vi "main.vi"() -> ()   [LabVIEW 2021]
uses:
  DIAS_Pyrometer/DIAS_Pyrometer.lvlib
  typedefs/MachineStates.ctl
  typedefs/GUIMsg.ctl
  7af14925-e625-4b71-82b2-5c041dc11c26.vi
  DIAS_Pyrometer/VIs/Server/TimeResp.ctl
  DIAS_Pyrometer/VIs/Server/PyrospotDat.ctl
  Library/TerminalDef.ctl
  Library/LibDan.lvlib
  Library/PromptWrite.vi
  Library/PassFailWrite.vi
  95fd1d63-83c7-47ba-856f-b2f4cd3ba726.vi
  DIAS_Pyrometer/SetTResp.vi
  DIAS_Pyrometer/SetEmi.vi
  5cd4da98-0f3d-48f1-83bd-2073b8292d09.vi
  Library/ErrorWrite.vi
  ec44e22e-e0b8-4ec3-9cb0-dd0efa94501a.vi
  4efa8287-acc7-4af3-aaf1-ea9888832d28.vi
  34df0790-2c42-4b95-90d0-b75bcdfa5c96.vi
  f4e94fa1-7f87-4e7c-9be3-fe64689eeddf.vi
  d668ad43-4b8f-4c4d-b9d8-3098d740c719.vi
  ba4263dd-0b88-4781-9c96-c1ae58dad5df.vi
  <vilib>/Utility/config.llb/Config Data RefNum.ctl
  <vilib>/Utility/config.llb/NI_LVConfig.lvlib
panel:
  out "LED_Serving":bool
  out "LED_Connected":bool
  in  "Stop":bool
  in  "Server_But":bool
  in  "Connect_But":bool
  out "Terminal":string
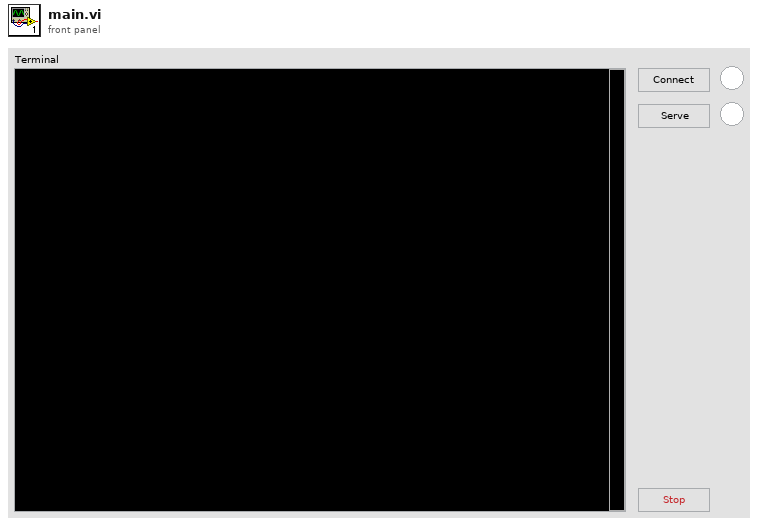
[diagram p1: front panel]
types:
  T1 = cluster{"Name":string, "Map":map{string, string}}
  T2 = typedef "DIAS_Pyrometer.lvlib/TimeResp.ctl" = u16
  T3 = typedef "LibDan.lvlib/TerminalDef.ctl" = cluster{"Terminal":cluster{"Data":string, "Prompt":string, "Output Refnum":refnum<vi>, "Input":string, "Input Refnum":refnum<vi>}, "TCP":cluster{"HostIP":string, "ServiceName":string, "Port":u16, "Timeout":i32, "TCP ID":refnum<k5>, "TCPConID":refnum<k5>, "Listening?":bool, "ClientCon?":bool}, "Config":cluster{"Path":path, "PathRef":T4, "NewFile?":bool, "Sections":cluster{"Name":string, "Map":map{string, string}}[]}}
  T4 = typedef "NI_LVConfig.lvlib/Config Data RefNum.ctl" = refnum<k1>
  T5 = typedef "DIAS_Pyrometer.lvlib/PyrospotDat.ctl" = cluster{"COM":u16, "Good":bool, "Address":i32, "Emissivity":sgl, "T95":T2, "Temp(K)":dbl, "Time":timestamp, "Laser":bool}
  T6 = typedef "MachineStates.ctl" = enum16{"NOP", "ProgInit", "PyroCon", "PyroDis", "Error", "SetPyro", "GetPyro", "ServerCon", "ServerDis", "ServeData", "ServerListen", "STOP"}
  T7 = typedef "GUIMsg.ctl" = cluster{T6, "exit?":bool}
  T8 = cluster{"Name":string, "Map":map{string, string}}[]
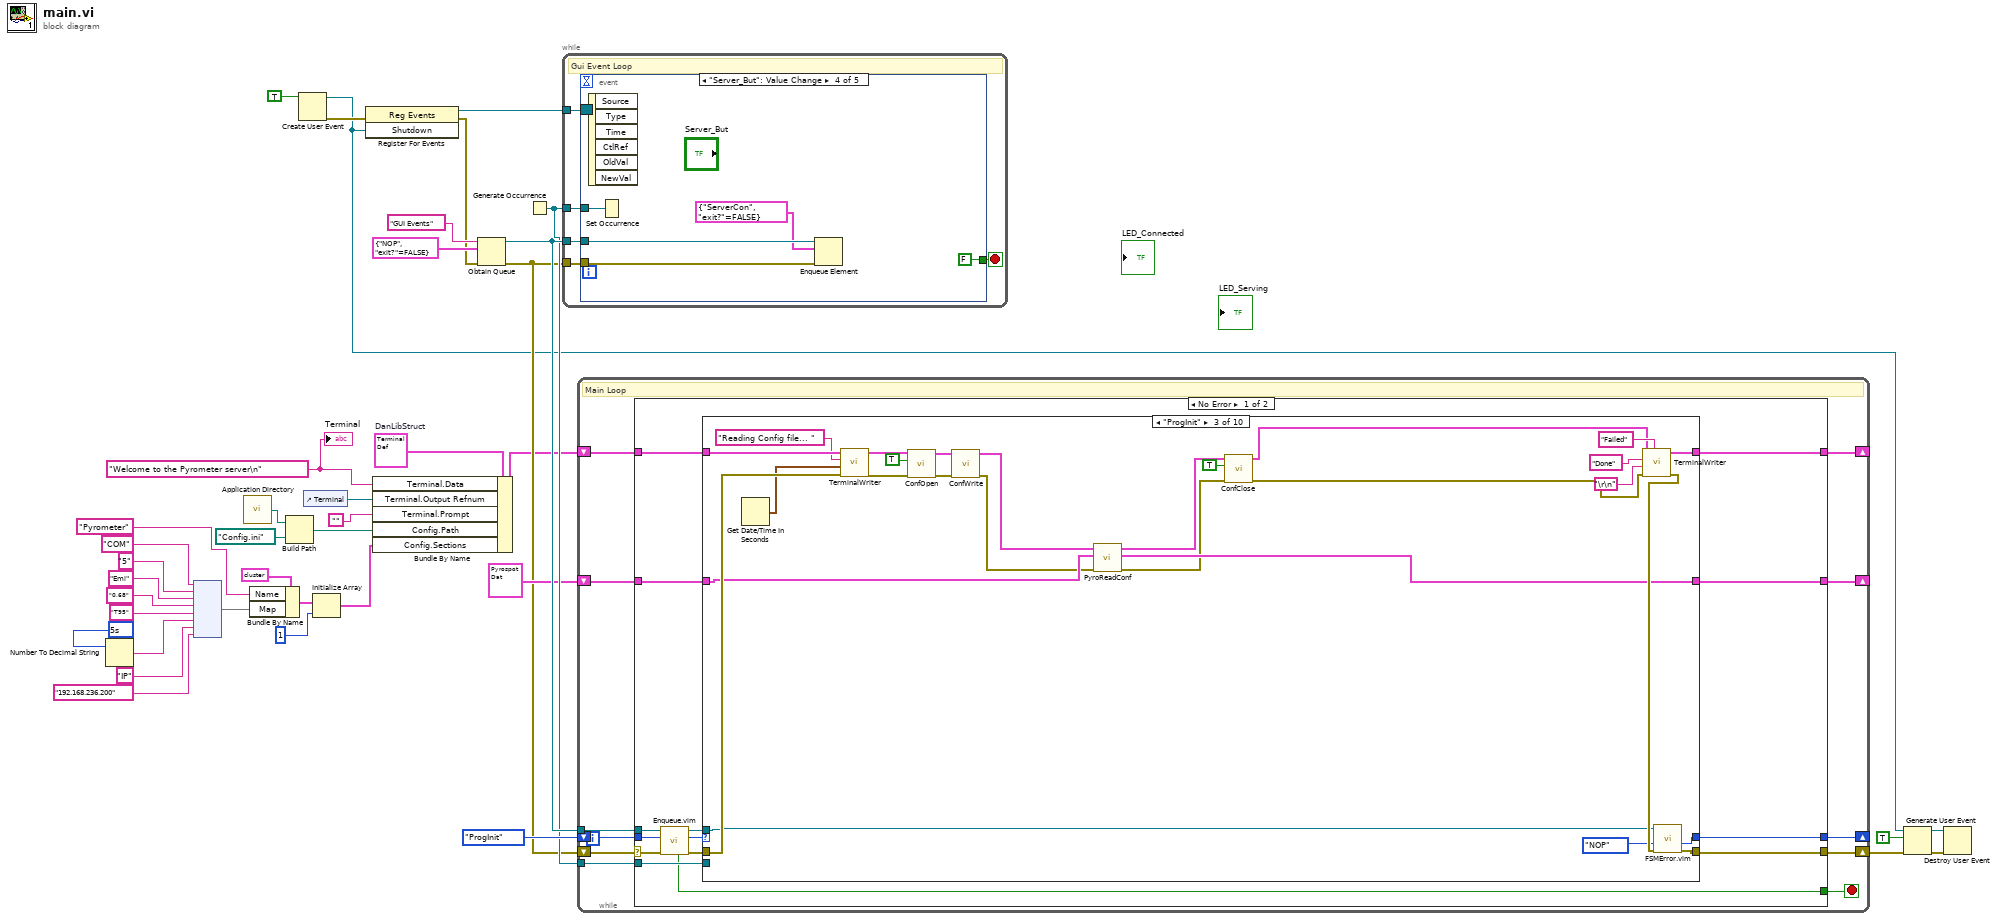
[diagram p0: block diagram]
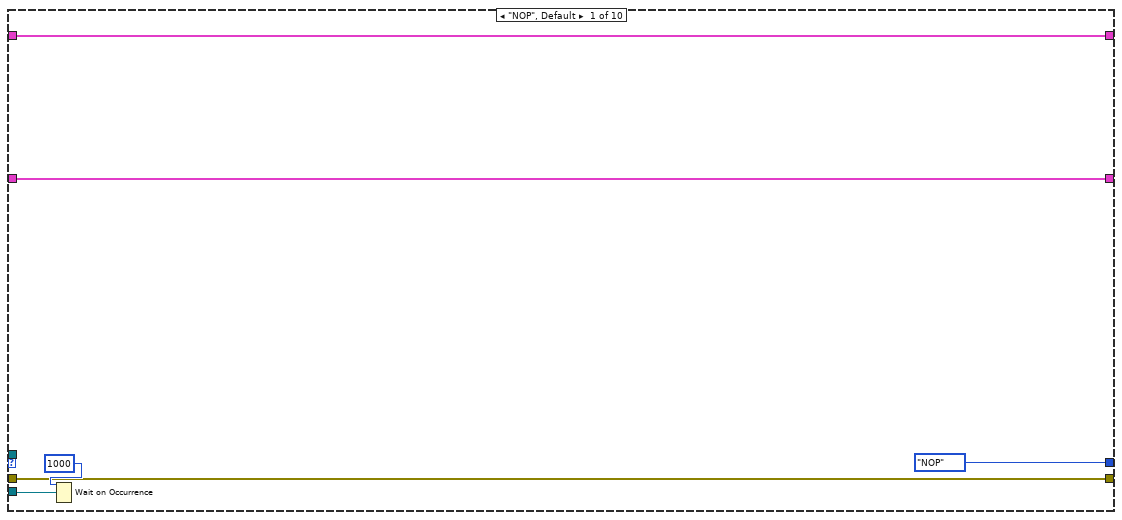
[diagram p2: hidden frame]
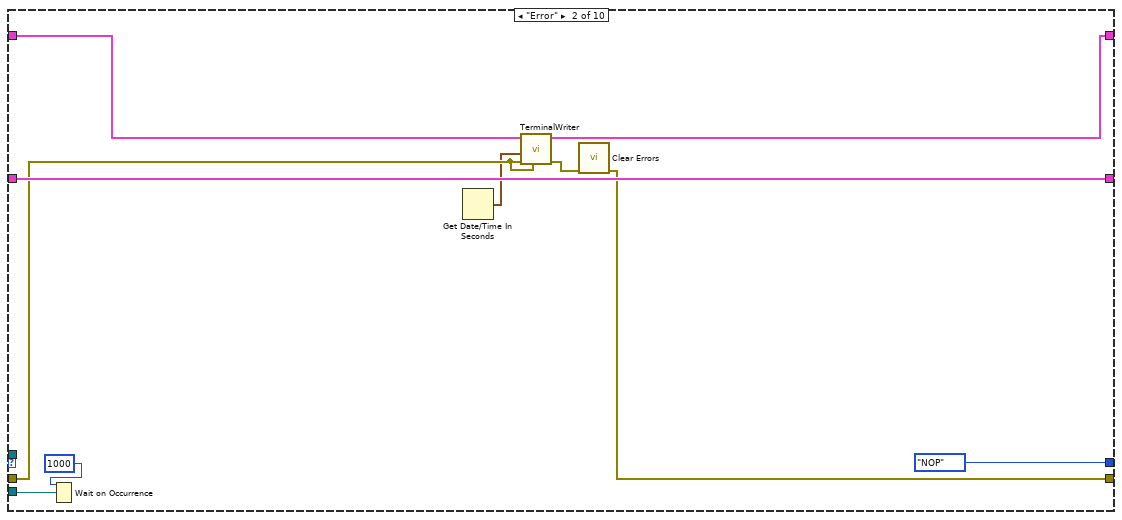
[diagram p3: hidden frame]
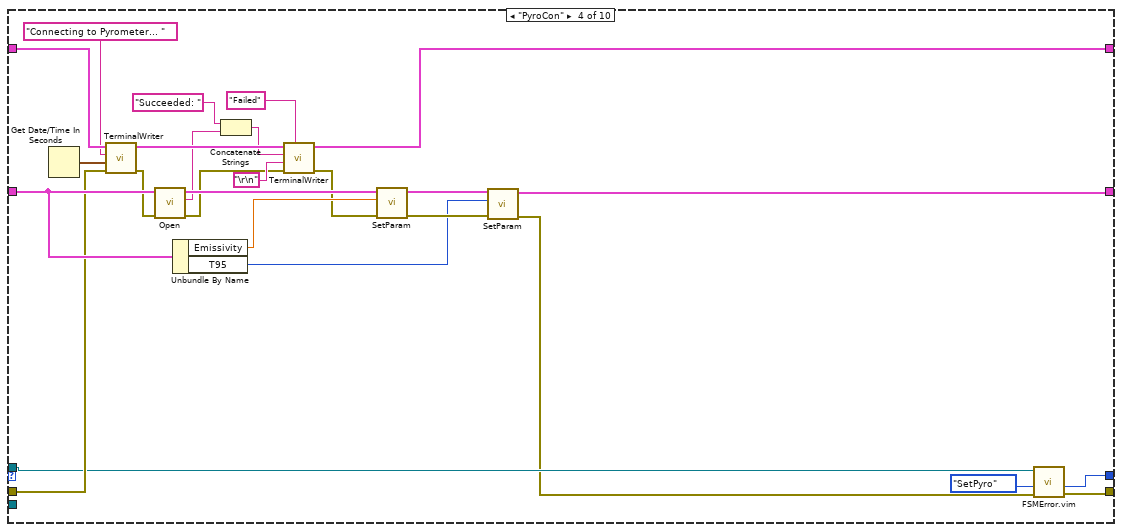
[diagram p4: hidden frame]
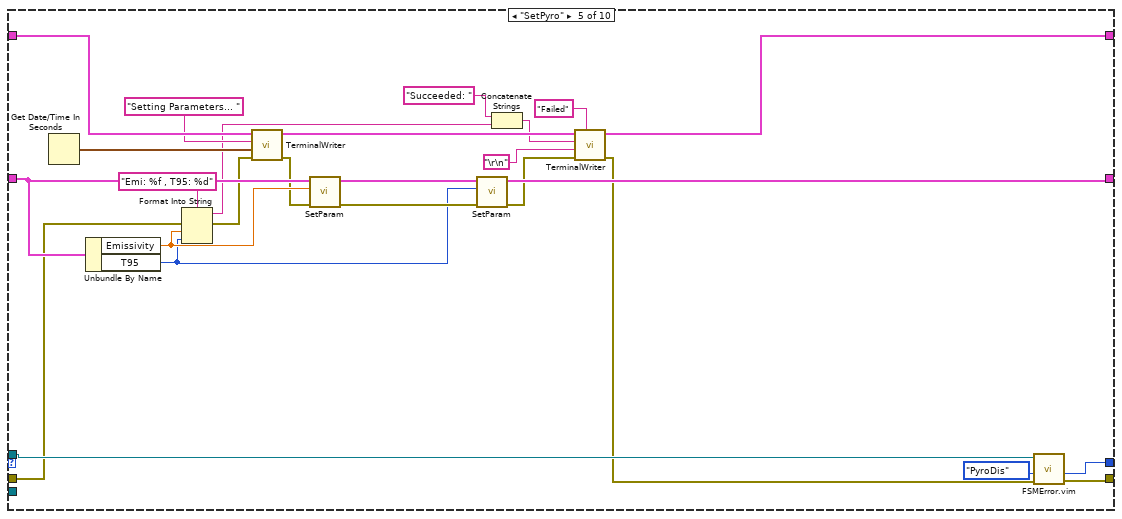
[diagram p5: hidden frame]
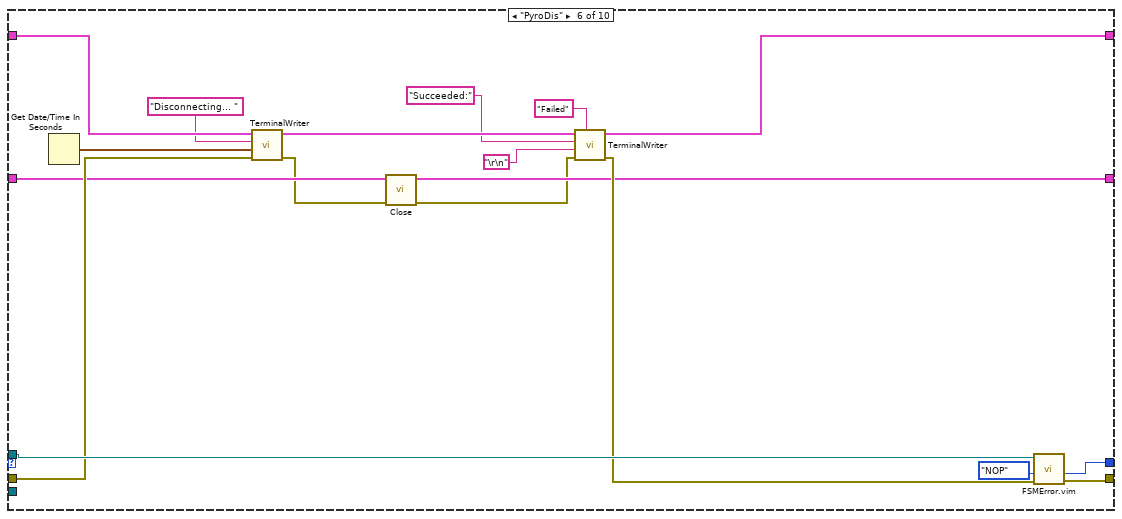
[diagram p6: hidden frame]
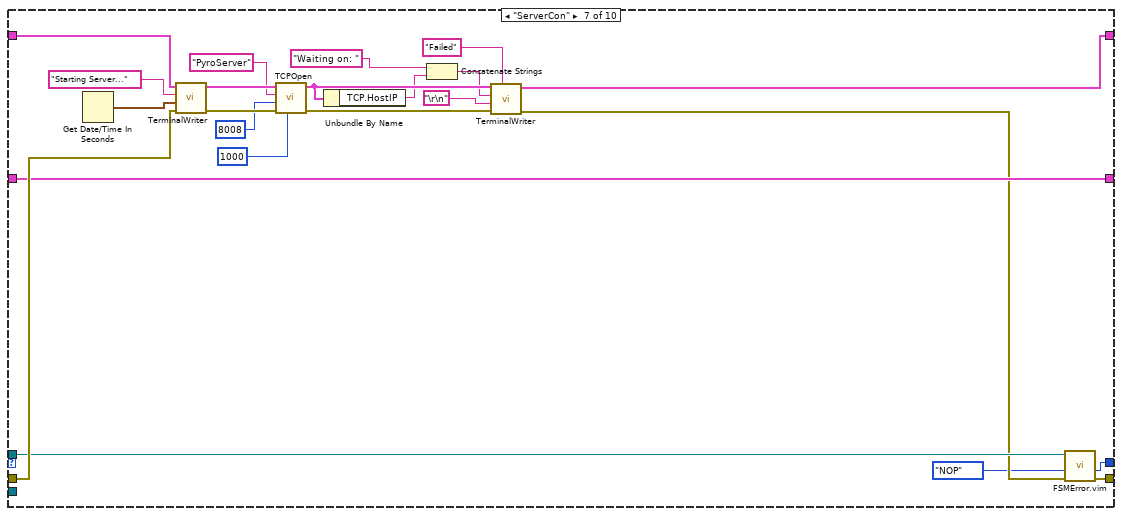
[diagram p7: hidden frame]
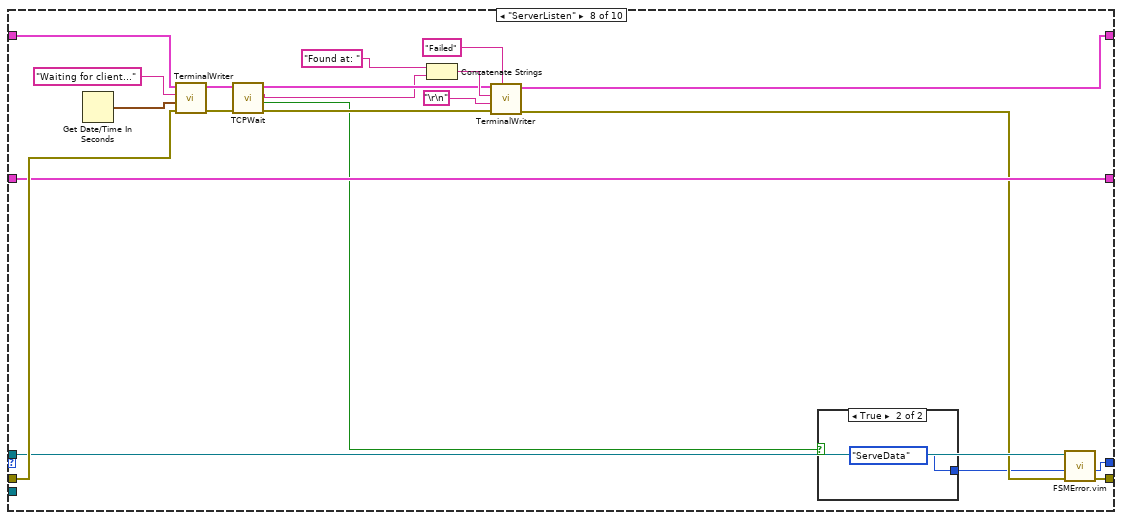
[diagram p8: hidden frame]
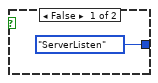
[diagram p9: hidden frame]
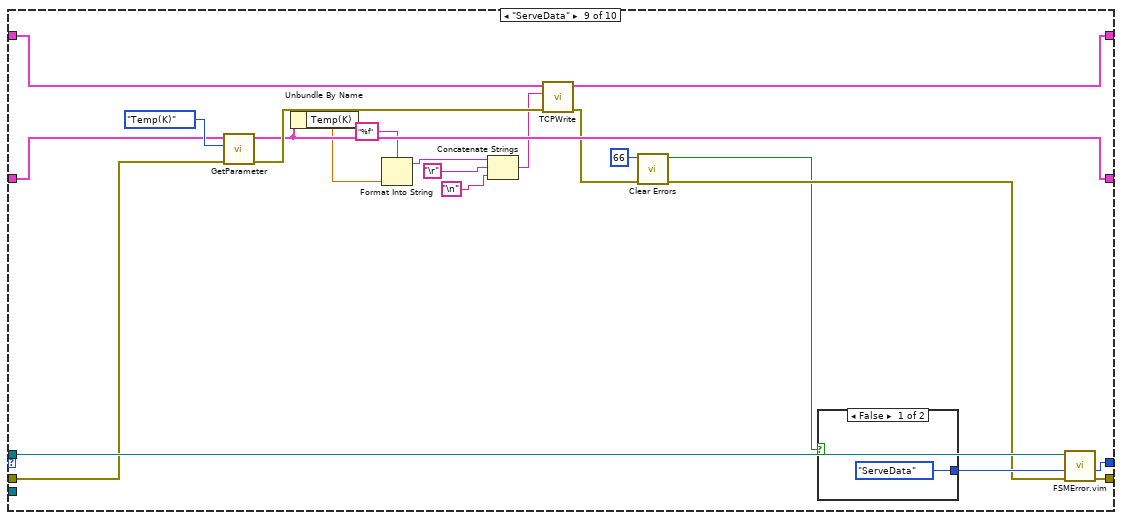
[diagram p10: hidden frame]
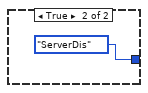
[diagram p11: hidden frame]
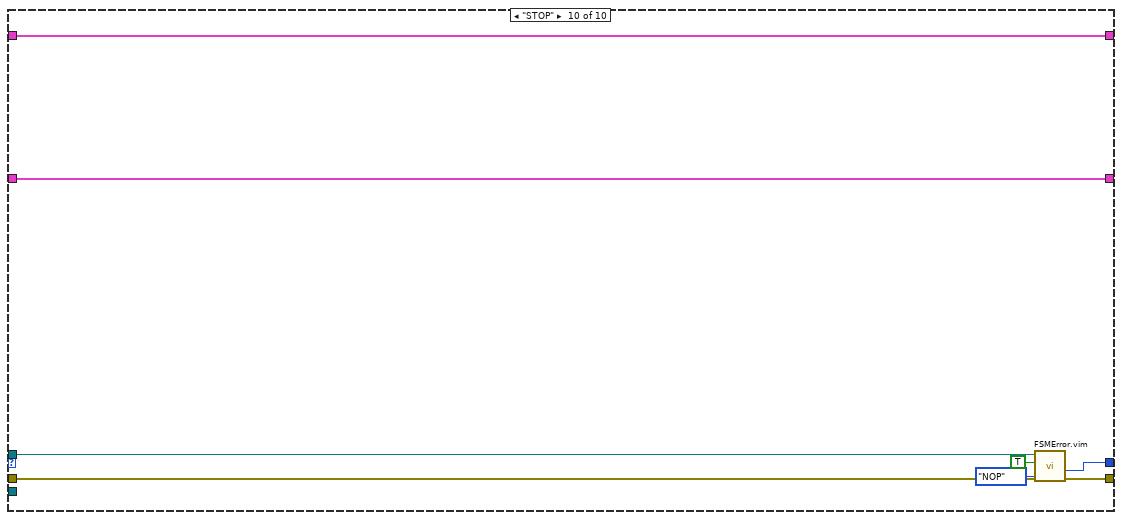
[diagram p12: hidden frame]
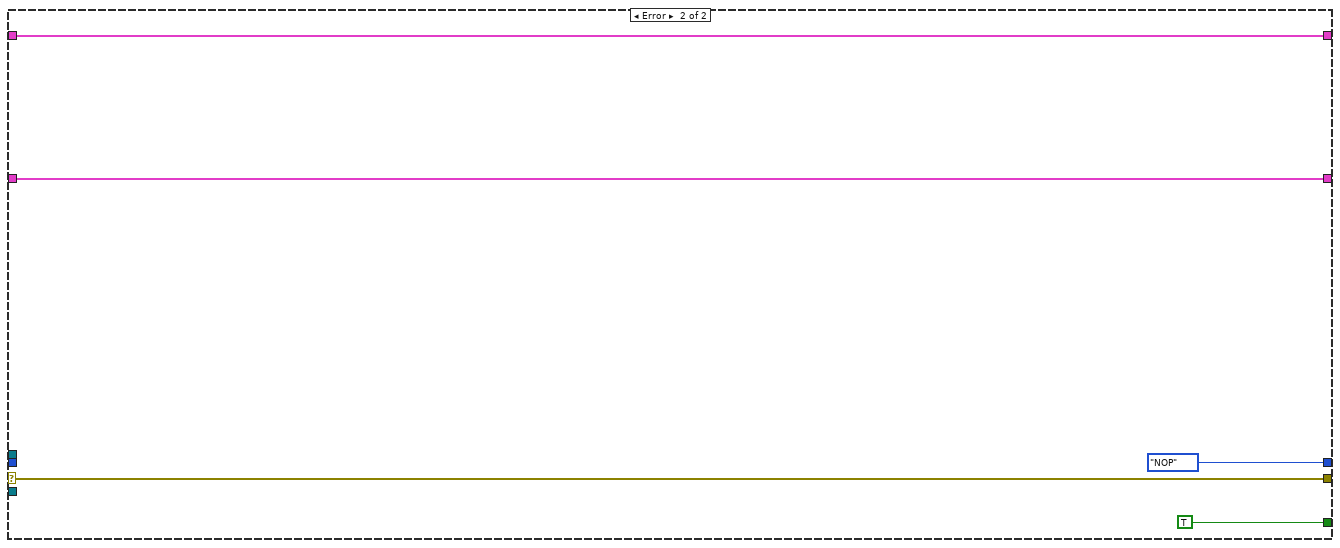
[diagram p13: hidden frame]
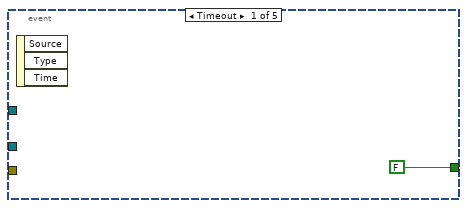
[diagram p14: hidden frame]
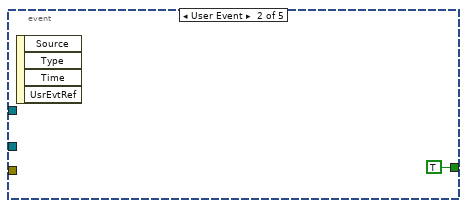
[diagram p15: hidden frame]
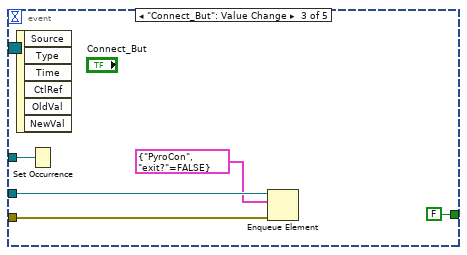
[diagram p16: hidden frame]
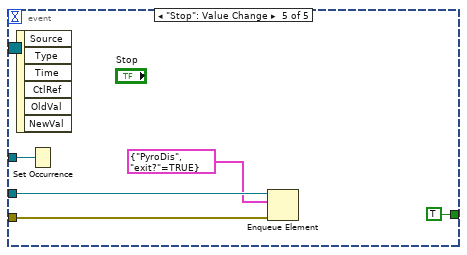
[diagram p17: hidden frame]
diagram:
  w10 = T2 21 items=["min/off"=0, "1ms"=10, "2ms"=11, "5ms"=12, "10ms"=13, "20ms"=14, "50ms"=15, "100ms"=16, "200ms"=17, "500ms"=18, "1s"=19, "2s"=20, "5s"=21, "10s"=22, "20s"=23, "50s"=24, "100s"=25] ("T95No")
  w20 = "Welcome to the Pyrometer server\n" ("Data")
  w23 = T3 {"Terminal"={"Data"="", "Prompt"="", "Output Refnum"=refnum, "Input"="", "Input Refnum"=refnum}, "TCP"={"HostIP"="", "ServiceName"="", "Port"=0, "Timeout"=0, "TCP ID"=refnum, "TCPConID"=refnum, "Listening?"=FALSE, "ClientCon?"=FALSE}, "Config"={"Path"=path "", "PathRef"=refnum, "NewFile?"=FALSE, "Sections"=[]}}  # DanLibStruct
  n1 = Number To Decimal String(number=w10) -> (decimal integer string=w9:string)  [unwired: 1 in]
  n2 = node("COM" ("key"), "5", "Emi", "0,68", "T95", w9, "IP", "192.168.236.200") -> (w4:map{string, string})
  n3 = call <vilib>:"Application Directory.vi"() -> ("Application Directory"=w17:path)
  n4 = Bundle By Name(cluster=T1 {"Name"="", "Map"={}} ("Cluster"), "Name"="Pyrometer", "Map"=w4) -> (w5:T1)
  n5 = Build Path(base path=w17, name or relative path=path "Config.ini") -> (appended path=w16:path)
  n6 = Create User Event(user event datatype=TRUE ("Shutdown")) -> (user event=w24:refnum<user-event>, error out=w32:errorcluster)  [unwired: 1 in]
  n7 = control-ref of="Terminal"() -> (w22:refnum<vi>)
  n8 = Initialize Array(w5, 1 ("dimension size")) -> (w2:T8)
  n9 = register-events(error in=w32, w24) -> (reference out=w26:refnum<event-registration>, error out=w25:errorcluster)  [unwired: 1 in]
  n10 = Bundle By Name(cluster=w23, "Terminal.Data"=w20, "Terminal.Output Refnum"=w22, "Terminal.Prompt"="", "Config.Path"=w16, "Config.Sections"=w2) -> (w21:T3)
  n11 = Obtain Queue(name (unnamed)="GUI Events", element data type=T7 {enum."NOP", "exit?"=FALSE}, error in (no error)=w25) -> (queue out=w36:refnum<queue>, error out=w31:errorcluster)  [unwired: 2 in, 1 out]
  n12 = Generate Occurrence() -> (w35:refnum<k4>)
  n13 = while {
    tunnel: w35 -> [w44]
    tunnel: w36 -> [w42]
    tunnel: w31 -> [w41]
    tunnel: w26 -> [w40]
    stop <- w43 stop-if-true
    # "Gui Event Loop"
    n14 = event shown="[3] \"Server_But\": Value Change" {
      selector: w40 -> [_ _ _ _ _]
      dyn-events: _ -> [_ _ _ _ _]
      timeout: _ -> [_ _ _ _ _]
      tunnel: w44 -> [_ _ w51 w56 w61]
      tunnel: [FALSE TRUE FALSE FALSE TRUE] -> w43
      tunnel: w42 -> [_ _ w50 w55 w60]
      tunnel: w41 -> [_ _ w49 w54 w59]
      event Timeout {
        n15 = event-data() -> ()  [unwired: 1 in, 3 out]
      }
      event User Event {
        n16 = event-data() -> ()  [unwired: 1 in, 4 out]
      }
      event "Connect_But": Value Change {
        n17 = event-data() -> ()  [unwired: 1 in, 6 out]
        n18 = Set Occurrence(w51) -> ()
        n19 = Enqueue Element(queue=w50, element=T7 {enum."PyroCon", "exit?"=FALSE}, error in (no error)=w49) -> ()  [unwired: 1 in, 3 out]
      }
      event "Server_But": Value Change {
        n20 = event-data() -> ()  [unwired: 1 in, 6 out]
        n21 = Set Occurrence(w56) -> ()
        n22 = Enqueue Element(queue=w55, element=T7 {enum."ServerCon", "exit?"=FALSE}, error in (no error)=w54) -> ()  [unwired: 1 in, 3 out]
      }
      event "Stop": Value Change {
        n23 = event-data() -> ()  [unwired: 1 in, 6 out]
        n24 = Set Occurrence(w61) -> ()
        n25 = Enqueue Element(queue=w60, element=T7 {enum."PyroDis", "exit?"=TRUE}, error in (no error)=w59) -> ()  [unwired: 1 in, 3 out]
      }
    }
  }
  n26 = while {
    tunnel: w36 -> [w70]
    shift-right: [w68] -> _
    shift-left: MachineStates."ProgInit" -> [w69]
    tunnel: w35 -> [w67]
    shift-right: [w65] -> _
    shift-left: T5 {"COM"=0, "Good"=FALSE, "Address"=0, "Emissivity"=0.0, "T95"=21, "Temp(K)"=0.0, "Time"=timestamp(0 s since 1904-01-01), "Laser"=FALSE} ("ClusterIn") -> [w66]
    shift-right: [w64] -> w30
    shift-left: w31 -> [w72]
    shift-right: [w62] -> _
    shift-left: w21 -> [w63]
    stop <- w71 stop-if-true
    # "Main Loop"
    n27 = case shown="No Error" w72 {
      selector: w72 -> [w81 w278]
      tunnel: [w77 TRUE] -> w71
      tunnel: w70 -> [w84 _]
      tunnel: w69 -> [w82 _]
      tunnel: [w86 MachineStates."NOP"] -> w68
      tunnel: w67 -> [w85 _]
      tunnel: w66 -> [w79 w279]
      tunnel: [w78 w279] -> w65
      tunnel: [w76 w278] -> w64
      tunnel: w63 -> [w75 w277]
      tunnel: [w74 w277] -> w62
      frame No Error {
        n28 = call "Enqueue.vim"("error in (no error)"=w81, "Variant"=w82, "queue In"=w84) -> ("error out"=w80:errorcluster, "Variant Out"=w83:T6, "queue out"=w73:refnum<queue>, "Exit?"=w77:bool)  [unwired: 5 in]
        n29 = case shown="\"ProgInit\"" w83 {
          tunnel: w73 -> [_ _ w118 w134 w168 w191 w204 w233 w266 w273]
          tunnel: w80 -> [w88 w94 w128 w141 w164 w187 w219 w240 w258 w275]
          tunnel: [MachineStates."NOP" MachineStates."NOP" w121 w133 w167 w190 w202 w231 w264 w272] -> w86
          tunnel: w85 -> [w91 w101 _ _ _ _ _ _ _ _]
          tunnel: w79 -> [w89 w99 w110 w154 w181 w185 w205 w234 w257 w276]
          tunnel: [w89 w99 w109 w151 w178 w184 w205 w234 w256 w276] -> w78
          tunnel: [w88 w95 w120 w132 w166 w189 w203 w232 w265 w271] -> w76
          tunnel: w75 -> [w87 w98 w129 w150 w177 w199 w221 w242 w261 w274]
          tunnel: [w87 w97 w125 w146 w173 w195 w206 w235 w262 w274] -> w74
          frame "NOP", Default {
            n30 = Wait on Occurrence(2:w91, 3:1000 ("ms timeout (-1)")) -> ()  [unwired: 1 in, 1 out]
          }
          frame "Error" {
            n31 = Wait on Occurrence(2:w101, 3:1000 ("ms timeout (-1)")) -> ()  [unwired: 1 in, 1 out]
            n32 = Get Date/Time In Seconds() -> (seconds since 1Jan1904=w93:timestamp)
            n33 = call-poly "TerminalWriter.vi"("Error to write"=w94, "error in"=w94, "time"=w93, "TerminalIn"=w98) -> ("error out"=w96:errorcluster, "TerminalOut"=w97:T3)  [unwired: 6 in]
            n34 = call <vilib>:"Clear Errors.vi"("error in (no error)"=w96) -> ("error out"=w95:errorcluster)  [unwired: 5 in, 1 out]
          }
          frame "ProgInit" {
            n35 = Get Date/Time In Seconds() -> (seconds since 1Jan1904=w127:timestamp)
            n36 = call-poly "TerminalWriter.vi"("error in"=w128, "time"=w127, "string"="Reading Config file... ", "TerminalIn"=w129) -> ("error out"=w115:errorcluster, "TerminalOut"=w116:T3)  [unwired: 6 in]
            n37 = call "ConfOpen.vi"("error in"=w115, "create file if necessary (T)"=TRUE, "StructIn"=w116) -> ("error out"=w112:errorcluster, "StructOut"=w113:T3)  [unwired: 6 in, 1 out]
            n38 = call "ConfWrite.vi"("error in"=w112, "StructIn"=w113) -> ("error out"=w108:errorcluster, "StructOut"=w111:T3)  [unwired: 8 in]
            n39 = call "PyroReadConf.vi"("error in"=w108, "PyroClusterIn"=w110, "StructIn"=w111) -> ("error out"=w107:errorcluster, "PyroClusterOut"=w109:T5, "StructOut"=w106:T3)  [unwired: 6 in]
            n40 = call "ConfClose.vi"("error in"=w107, "Write?"=TRUE, "StructIn"=w106) -> ("error out"=w103:errorcluster, "StructOut"=w104:T3)  [unwired: 7 in]
            n41 = call-poly "TerminalWriter.vi"("FailString"="Failed", "error in"=w103, "End"="\r\n", "PassString"="Done" ("string"), "TerminalIn"=w104) -> ("error out"=w119:errorcluster, "TerminalOut"=w125:T3)  [unwired: 5 in]
            n42 = call "FSMError.vim"("error"=w119, "State"=MachineStates."NOP", "queue In"=w118) -> ("error IO"=w120:errorcluster, "stateout"=w121:T6)  [unwired: 6 in, 1 out]
          }
          frame "PyroCon" {
            n43 = Get Date/Time In Seconds() -> (seconds since 1Jan1904=w148:timestamp)
            n44 = call-poly "TerminalWriter.vi"("error in"=w141, "time"=w148, "string"="Connecting to Pyrometer... ", "TerminalIn"=w150) -> ("error out"=w140:errorcluster, "TerminalOut"=w147:T3)  [unwired: 6 in]
            n45 = call "Open.vi"("error in (no error)"=w140, "ClusterIn"=w154) -> ("error out"=w139:errorcluster, "name out"=w136:string, "ClusterOut"=w155:T5)  [unwired: 6 in, 1 out]
            n46 = Unbundle By Name(w154) -> ("Emissivity"=w143:sgl, "T95"=w142:T2)
            n47 = Concatenate Strings("Succeeded: " ("string"), w136) -> (w135:string)
            n48 = call-poly "TerminalWriter.vi"("FailString"="Failed" ("string"), "error in"=w139, "End"="\r\n", "PassString"=w135, "TerminalIn"=w147) -> ("error out"=w138:errorcluster, "TerminalOut"=w146:T3)  [unwired: 5 in]
            n49 = call-poly "SetParam.vi"("error in"=w138, "emi"=w143, "ClusterIn"=w155) -> ("errorout"=w152:errorcluster, "ClusterOut"=w153:T5)  [unwired: 7 in]
            n50 = call-poly "SetParam.vi"("error in"=w152, "T95"=w142, "ClusterIn"=w153) -> ("errorout"=w131:errorcluster, "ClusterOut"=w151:T5)  [unwired: 7 in]
            n51 = call "FSMError.vim"("error"=w131, "State"=MachineStates."SetPyro", "queue In"=w134) -> ("error IO"=w132:errorcluster, "stateout"=w133:T6)  [unwired: 6 in, 1 out]
          }
          frame "SetPyro" {
            n52 = Get Date/Time In Seconds() -> (seconds since 1Jan1904=w175:timestamp)
            n53 = Unbundle By Name(w181) -> ("Emissivity"=w160:sgl, "T95"=w159:T2)
            n54 = Format Into String(format string="Emi: %f , T95: %d", error in=w164, w160, w159) -> (resulting string=w156:string, error out=w158:errorcluster)  [unwired: 1 in]
            n55 = call-poly "TerminalWriter.vi"("error in"=w158, "time"=w175, "string"="Setting Parameters... ", "TerminalIn"=w177) -> ("error out"=w157:errorcluster, "TerminalOut"=w174:T3)  [unwired: 6 in]
            n56 = call-poly "SetParam.vi"("error in"=w157, "emi"=w160, "ClusterIn"=w181) -> ("errorout"=w179:errorcluster, "ClusterOut"=w180:T5)  [unwired: 7 in]
            n57 = call-poly "SetParam.vi"("error in"=w179, "T95"=w159, "ClusterIn"=w180) -> ("errorout"=w163:errorcluster, "ClusterOut"=w178:T5)  [unwired: 7 in]
            n58 = Concatenate Strings("Succeeded: " ("string"), w156) -> (w169:string)
            n59 = call-poly "TerminalWriter.vi"("FailString"="Failed" ("string"), "error in"=w163, "End"="\r\n", "PassString"=w169, "TerminalIn"=w174) -> ("error out"=w162:errorcluster, "TerminalOut"=w173:T3)  [unwired: 5 in]
            n60 = call "FSMError.vim"("error"=w162, "State"=MachineStates."PyroDis", "queue In"=w168) -> ("error IO"=w166:errorcluster, "stateout"=w167:T6)  [unwired: 6 in, 1 out]
          }
          frame "PyroDis" {
            n61 = Get Date/Time In Seconds() -> (seconds since 1Jan1904=w197:timestamp)
            n62 = call-poly "TerminalWriter.vi"("error in"=w187, "time"=w197, "string"="Disconnecting... ", "TerminalIn"=w199) -> ("error out"=w183:errorcluster, "TerminalOut"=w196:T3)  [unwired: 6 in]
            n63 = call "Close.vi"("error in (no error)"=w183, "ClusterIn"=w185) -> ("error out"=w182:errorcluster, "ClusterOut"=w184:T5)  [unwired: 8 in]
            n64 = call-poly "TerminalWriter.vi"("FailString"="Failed" ("string"), "error in"=w182, "End"="\r\n", "PassString"="Succeeded:" ("string"), "TerminalIn"=w196) -> ("error out"=w186:errorcluster, "TerminalOut"=w195:T3)  [unwired: 5 in]
            n65 = call "FSMError.vim"("error"=w186, "State"=MachineStates."NOP", "queue In"=w191) -> ("error IO"=w189:errorcluster, "stateout"=w190:T6)  [unwired: 6 in, 1 out]
          }
          frame "ServerCon" {
            n66 = Get Date/Time In Seconds() -> (seconds since 1Jan1904=w220:timestamp)
            n67 = call-poly "TerminalWriter.vi"("error in"=w219, "time"=w220, "string"="Starting Server...", "TerminalIn"=w221) -> ("error out"=w218:errorcluster, "TerminalOut"=w217:T3)  [unwired: 6 in]
            n68 = call "TCPOpen.vi"("timeout"=1000, "error in"=w218, "port"=u16 8008, "service name"="PyroServer", "StructIn"=w217) -> ("error out"=w213:errorcluster, "StructOut"=w212:T3)  [unwired: 5 in]
            n69 = Unbundle By Name(w212) -> ("TCP.HostIP"=w211:string)
            n70 = Concatenate Strings("Waiting on: " ("string"), w211) -> (w209:string)
            n71 = call-poly "TerminalWriter.vi"("FailString"="Failed", "error in"=w213, "End"="\r\n", "PassString"=w209, "TerminalIn"=w212) -> ("error out"=w201:errorcluster, "TerminalOut"=w206:T3)  [unwired: 5 in]
            n72 = call "FSMError.vim"("error"=w201, "State"=MachineStates."NOP", "queue In"=w204) -> ("error IO"=w203:errorcluster, "stateout"=w202:T6)  [unwired: 6 in, 1 out]
          }
          frame "ServerListen" {
            n73 = Get Date/Time In Seconds() -> (seconds since 1Jan1904=w241:timestamp)
            n74 = call-poly "TerminalWriter.vi"("error in"=w240, "time"=w241, "string"="Waiting for client...", "TerminalIn"=w242) -> ("error out"=w227:errorcluster, "TerminalOut"=w229:T3)  [unwired: 6 in]
            n75 = call "TCPWait.vi"("error in"=w227, "StructIn"=w229) -> ("error out"=w226:errorcluster, "Connected"=w224:bool, "remote address"=w225:string, "StructOut"=w228:T3)  [unwired: 6 in]
            n76 = Concatenate Strings("Found at: " ("string"), w225) -> (w238:string)
            n77 = call-poly "TerminalWriter.vi"("FailString"="Failed", "error in"=w226, "End"="\r\n", "PassString"=w238, "TerminalIn"=w228) -> ("error out"=w230:errorcluster, "TerminalOut"=w235:T3)  [unwired: 5 in]
            n78 = case shown="True" w224 {
              tunnel: [MachineStates."ServerListen" ("State") MachineStates."ServeData" ("State")] -> w223
              frame False {
              }
              frame True {
              }
            }
            n79 = call "FSMError.vim"("error"=w230, "State"=w223, "queue In"=w233) -> ("error IO"=w232:errorcluster, "stateout"=w231:T6)  [unwired: 6 in, 1 out]
          }
          frame "ServeData" {
            n80 = call "GetParameter.vi"("error in"=w258, "Parameter"=enum16{"Emissivity", "T95", "Temp(K)"}."Temp(K)", "ClusterIn"=w257) -> ("errorout"=w259:errorcluster, "ClusterOut"=w256:T5)  [unwired: 7 in]
            n81 = Unbundle By Name(w256) -> ("Temp(K)"=w255:dbl)
            n82 = Format Into String(format string="%f", w255) -> (resulting string=w253:string)  [unwired: 2 in, 1 out]
            n83 = Concatenate Strings(w253, "\r", "\n") -> (w250:string)
            n84 = call "TCPWrite.vi"("error in"=w259, "data in"=w250, "StructIn"=w261) -> ("error out"=w248:errorcluster, "StructOut"=w262:T3)  [unwired: 6 in, 1 out]
            n85 = call <vilib>:"Clear Errors.vi"("error in (no error)"=w248, "specific error code to clear (0: all)"=66) -> ("error out"=w247:errorcluster, "specific error cleared?"=w246:bool)  [unwired: 4 in]
            n86 = case shown="False" w246 {
              tunnel: [MachineStates."ServeData" ("State") MachineStates."ServerDis" ("State")] -> w263
              frame False {
              }
              frame True {
              }
            }
            n87 = call "FSMError.vim"("error"=w247, "State"=w263, "queue In"=w266) -> ("error IO"=w265:errorcluster, "stateout"=w264:T6)  [unwired: 6 in, 1 out]
          }
          frame "STOP" {
            n88 = call "FSMError.vim"("error"=w275, "State"=MachineStates."NOP", "Exit?"=TRUE, "queue In"=w273) -> ("error IO"=w271:errorcluster, "stateout"=w272:T6)  [unwired: 5 in, 1 out]
          }
        }
      }
      frame Error {
      }
    }
  }
  n89 = Generate User Event(user event=w24, event data cluster=TRUE ("event data"), error in=w30) -> (user event out=w28:refnum<user-event>, error out=w27:errorcluster)  [unwired: 1 in]
  n90 = Destroy User Event(user event=w28, error in=w27) -> ()  [unwired: 1 out]
  "Terminal" <- w20
